vi "XNET Database Close (Database).vi"(0 "database in":refnum<k21>, 5 "close all? (true)":bool=TRUE, 11 "error in (no error)":errorcluster) -> (15 "error out":errorcluster)   [LabVIEW 2018]
doc: "Closes a database object (or all objects in the database)."
uses:
  nixlvapi.dll
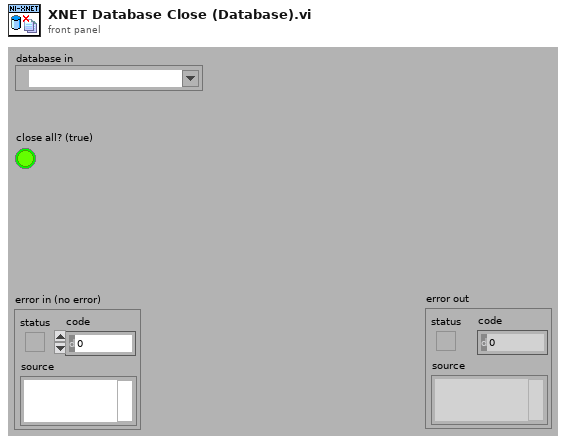
[diagram p1: front panel]
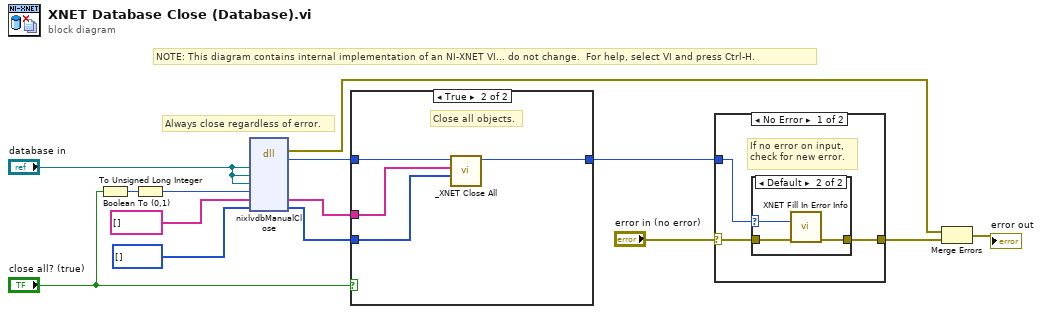
[diagram p0: block diagram]
diagram:
  # "Always close regardless of error."
  # "NOTE: This diagram contains internal implementation of an NI-XNET VI... do not change.  For help, select VI and press Ctrl-H."
  n1 = Boolean To (0,1)(Boolean="close all? (true)") -> (0, 1=w12:i16)
  n2 = To Unsigned Long Integer(number=w12) -> (unsigned 32bit integer=w10:u32)
  n3 = dll-call lib="nixlvapi.*" fn="nixlvdbManualClose"("reference"="database in", "lvObjectName"="database in", "refObjPtr"="database in", "closeAll"=w10, "allNames"=string[] [] ("array of alias"), "allClasses"=u32[] [] ("array of alias")) -> (error out=w1:errorcluster, "return type"=w7:i32, "allNames"=w6:string[], "allClasses"=w5:u32[])  [unwired: 5 in, 3 out]
  n4 = case shown="True" "close all? (true)" {
    tunnel: w6 -> [_ w17]
    tunnel: w5 -> [_ w16]
    tunnel: w7 -> [w15 w19]
    tunnel: [w15 w18] -> w3
    frame False {
      # "For a single object (close all? false),\nthe previous call closed in driver and LV."
    }
    frame True {
      # "Close all objects."
      n5 = call "_XNET Close All.vi"("all classes"=w16, "all names"=w17, "status code in"=w19) -> ("status code out"=w18:i32)  [unwired: 7 out]
    }
  }
  n6 = case shown="No Error" "error in (no error)" {
    selector: "error in (no error)" -> [w21 w27]
    tunnel: [w22 w27] -> w14
    tunnel: w3 -> [w20 _]
    frame No Error {
      # "If no error on input, \ncheck for new error."
      n7 = case shown="Default" w20 {
        selector: w20 -> [_ w24]
        tunnel: w21 -> [w23 w25]
        tunnel: [w23 w26] -> w22
        frame 0 {
        }
        frame Default {
          n8 = call "XNET Fill In Error Info.vi"("status code"=w24, "error in"=w25) -> ("error out"=w26:errorcluster)  [unwired: 13 out]
        }
      }
    }
    frame Error {
    }
  }
  n9 = Merge Errors(w1, w14) -> (→"error out":errorcluster)
